vi "slider timer .vi"(6 "interval (sec)":dbl=nan, 7 "action":T1, 11 "timer ref":refnum<vi>) -> (1 "tic":bool, 2 "tic state":enum16{"knock-knock", "none"}(ring), 3 "timer out":refnum<vi>)   [LabVIEW 2015]
uses:
  countdown control.ctl
  Q - not nan -- real.vi
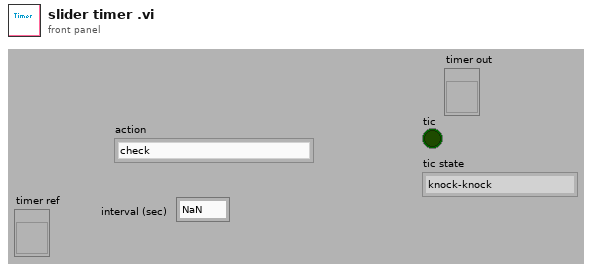
[diagram p1: front panel]
types:
  T1 = typedef "countdown control.ctl" = enum16{"check", "start", "reset cont", "stop", "reset once"}
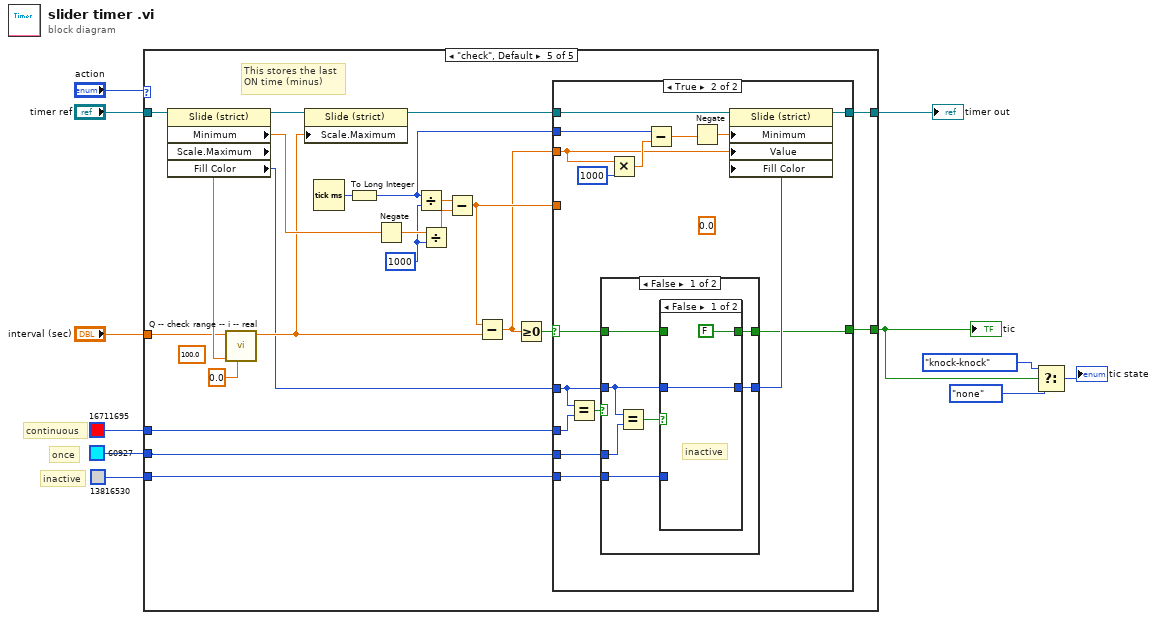
[diagram p0: block diagram]
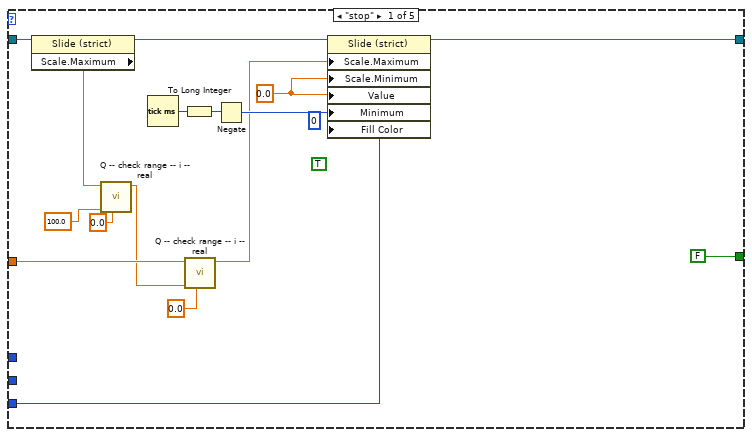
[diagram p2: hidden frame]
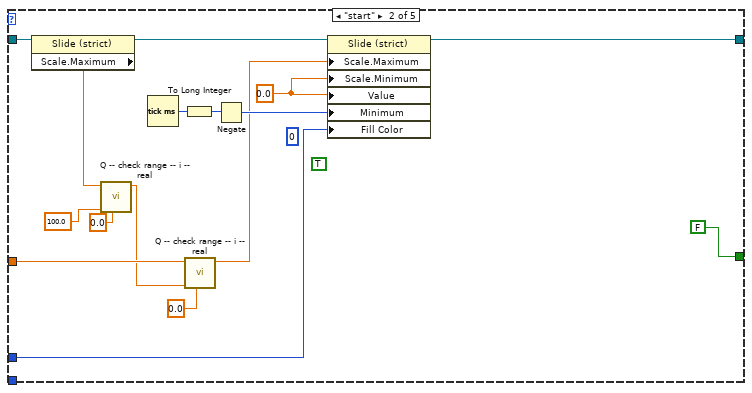
[diagram p3: hidden frame]
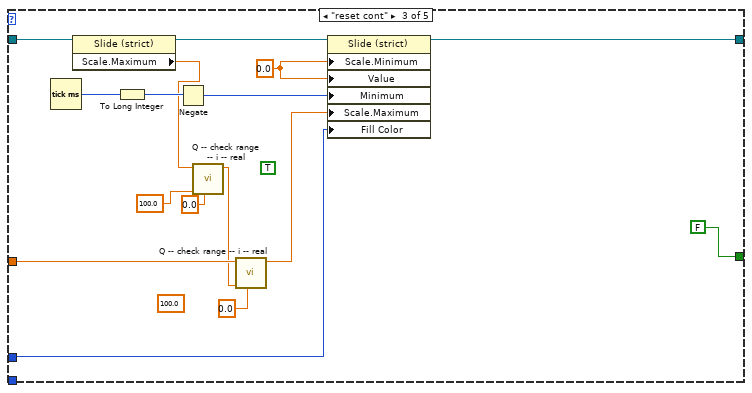
[diagram p4: hidden frame]
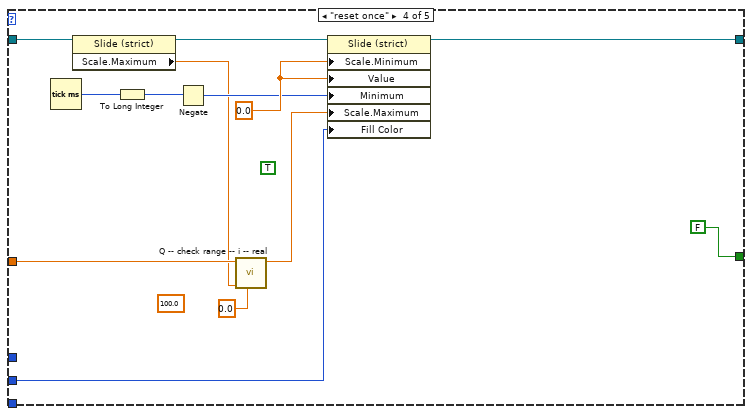
[diagram p5: hidden frame]
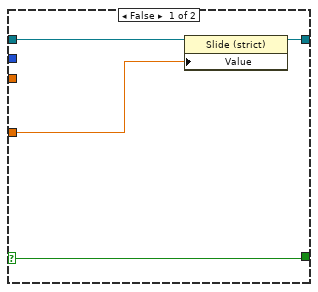
[diagram p6: hidden frame]
diagram:
  # "inactive"
  # "once"
  # "continuous"
  n1 = case shown="\"check\", Default" "action" {
    tunnel: "interval (sec)" -> [w21 w37 w50 w63 w81]
    tunnel: [FALSE FALSE FALSE FALSE w95] -> w9
    tunnel: [w25 w41 w57 w70 w91] -> w5
    tunnel: "timer ref" -> [w18 w34 w53 w66 w93]
    tunnel: u32 60927 -> [_ _ _ w60 w74]
    tunnel: u32 16711695 -> [_ w28 w48 _ w76]
    tunnel: u32 13816530 -> [w12 _ _ _ w73]
    frame "stop" {
      (unwired) u32 0 ("Fill Color")
      (unwired) TRUE
      w26 = 0.0 ("Thermometer")
      n2 = property class="Slide (strict)"(reference=w18) -> (reference out=w17:refnum<vi>, "Scale.Maximum"=w15:dbl)  [unwired: 1 in, 1 out]
      n3 = call "Q -- check range -- i -- real.vi"("lower"=0.0, "default"=100.0 ("t"), "number"=w15) -> ("number in range"=w13:dbl)  [unwired: 6 in, 2 out]
      n4 = Tick Count (ms)() -> (millisecond timer value=w23:u32)
      n5 = To Long Integer(number=w23) -> (32bit integer=w22:i32)
      n6 = call "Q -- check range -- i -- real.vi"("lower"=0.0, "default"=w13, "number"=w21) -> ("number in range"=w19:dbl)  [unwired: 6 in, 2 out]
      n7 = Negate(x=w22) -> (-x=w24:i32)
      n8 = property class="Slide (strict)"(reference=w17, "Scale.Maximum"=w19, "Scale.Minimum"=w26, "Value"=w26, "Minimum"=w24, "Fill Color"=w12) -> (reference out=w25:refnum<vi>)  [unwired: 1 in, 1 out]
    }
    frame "start" {
      (unwired) u32 0 ("Fill Color")
      (unwired) TRUE
      w42 = 0.0 ("Thermometer")
      n9 = property class="Slide (strict)"(reference=w34) -> (reference out=w33:refnum<vi>, "Scale.Maximum"=w31:dbl)  [unwired: 1 in, 1 out]
      n10 = call "Q -- check range -- i -- real.vi"("lower"=0.0, "default"=100.0 ("t"), "number"=w31) -> ("number in range"=w29:dbl)  [unwired: 6 in, 2 out]
      n11 = Tick Count (ms)() -> (millisecond timer value=w39:u32)
      n12 = To Long Integer(number=w39) -> (32bit integer=w38:i32)
      n13 = call "Q -- check range -- i -- real.vi"("lower"=0.0, "default"=w29, "number"=w37) -> ("number in range"=w35:dbl)  [unwired: 6 in, 2 out]
      n14 = Negate(x=w38) -> (-x=w40:i32)
      n15 = property class="Slide (strict)"(reference=w33, "Scale.Maximum"=w35, "Scale.Minimum"=w42, "Value"=w42, "Minimum"=w40, "Fill Color"=w28) -> (reference out=w41:refnum<vi>)  [unwired: 1 in, 1 out]
    }
    frame "reset cont" {
      (unwired) 100.0 ("t")
      (unwired) TRUE
      w58 = 0.0 ("Thermometer")
      n16 = Tick Count (ms)() -> (millisecond timer value=w55:u32)
      n17 = property class="Slide (strict)"(reference=w53) -> (reference out=w52:refnum<vi>, "Scale.Maximum"=w44:dbl)  [unwired: 1 in, 1 out]
      n18 = To Long Integer(number=w55) -> (32bit integer=w54:i32)
      n19 = Negate(x=w54) -> (-x=w56:i32)
      n20 = call "Q -- check range -- i -- real.vi"("lower"=0.0, "default"=100.0 ("t"), "number"=w44) -> ("number in range"=w45:dbl)  [unwired: 6 in, 2 out]
      n21 = call "Q -- check range -- i -- real.vi"("lower"=0.0, "default"=w45, "number"=w50) -> ("number in range"=w49:dbl)  [unwired: 6 in, 2 out]
      n22 = property class="Slide (strict)"(reference=w52, "Scale.Minimum"=w58, "Value"=w58, "Minimum"=w56, "Scale.Maximum"=w49, "Fill Color"=w48) -> (reference out=w57:refnum<vi>)  [unwired: 1 in, 1 out]
    }
    frame "reset once" {
      (unwired) 100.0 ("t")
      (unwired) TRUE
      w71 = 0.0 ("Thermometer")
      n23 = Tick Count (ms)() -> (millisecond timer value=w68:u32)
      n24 = property class="Slide (strict)"(reference=w66) -> (reference out=w65:refnum<vi>, "Scale.Maximum"=w61:dbl)  [unwired: 1 in, 1 out]
      n25 = To Long Integer(number=w68) -> (32bit integer=w67:i32)
      n26 = Negate(x=w67) -> (-x=w69:i32)
      n27 = call "Q -- check range -- i -- real.vi"("lower"=0.0, "default"=w61, "number"=w63) -> ("number in range"=w62:dbl)  [unwired: 6 in, 2 out]
      n28 = property class="Slide (strict)"(reference=w65, "Scale.Minimum"=w71, "Value"=w71, "Minimum"=w69, "Scale.Maximum"=w62, "Fill Color"=w60) -> (reference out=w70:refnum<vi>)  [unwired: 1 in, 1 out]
    }
    frame "check", Default {
      (unwired) 100.0 ("t")
      w77 = 1000
      # "This stores the last \nON time (minus)"
      n29 = property class="Slide (strict)"(reference=w93) -> (reference out=w85:refnum<vi>, "Minimum"=w87:dbl, "Scale.Maximum"=w82:dbl, "Fill Color"=w75:u32)  [unwired: 1 in, 1 out]
      n30 = call "Q -- check range -- i -- real.vi"("lower"=0.0, "default"=w82, "number"=w81) -> ("number in range"=w80:dbl)  [unwired: 6 in, 2 out]
      n31 = property class="Slide (strict)"(reference=w85, "Scale.Maximum"=w80) -> (reference out=w84:refnum<vi>)  [unwired: 1 in, 1 out]
      n32 = Tick Count (ms)() -> (millisecond timer value=w79:u32)
      n33 = To Long Integer(number=w79) -> (32bit integer=w78:i32)
      n34 = Negate(x=w87) -> (-x=w86:dbl)
      n35 = Divide(x=w78, y=w77) -> (x/y=w94:dbl)
      n36 = Divide(x=w86, y=w77) -> (x/y=w92:dbl)
      n37 = Subtract(x=w94, y=w92) -> (x-y=w90:dbl)
      n38 = Subtract(x=w90, y=w80) -> (x-y=w88:dbl)
      n39 = Greater Or Equal To 0?(x=w88) -> (x >= 0?=w89:bool)
      n40 = case shown="True" w89 {
        selector: w89 -> [w99 w102]
        tunnel: [w99 w101] -> w95
        tunnel: w90 -> [w98 _]
        tunnel: w84 -> [w96 w115]
        tunnel: w78 -> [_ w111]
        tunnel: [w97 w114] -> w91
        tunnel: w88 -> [_ w108]
        tunnel: w75 -> [_ w105]
        tunnel: w76 -> [_ w107]
        tunnel: w74 -> [_ w103]
        tunnel: w73 -> [_ w100]
        frame False {
          n41 = property class="Slide (strict)"(reference=w96, "Value"=w98) -> (reference out=w97:refnum<vi>)  [unwired: 1 in, 1 out]
        }
        frame True {
          (unwired) 0.0 ("Value")
          n42 = Equal?(x=w105, y=w107) -> (x = y?=w106:bool)
          n43 = case shown="False" w106 {
            tunnel: [w118 w128] -> w104
            tunnel: w105 -> [w116 w128]
            tunnel: w103 -> [w122 _]
            tunnel: w102 -> [w120 w127]
            tunnel: [w119 w127] -> w101
            tunnel: w100 -> [w117 _]
            frame False {
              n44 = Equal?(x=w116, y=w122) -> (x = y?=w121:bool)
              n45 = case shown="False" w121 {
                tunnel: [FALSE w126] -> w119
                tunnel: w120 -> [_ w126]
                tunnel: [w123 w125] -> w118
                tunnel: w117 -> [_ w125]
                tunnel: w116 -> [w123 _]
                frame False {
                  # "inactive"
                }
                frame True {
                  # "once"
                }
              }
            }
            frame True {
              # "continuous"
            }
          }
          n46 = Multiply(x=w108, y=1000) -> (x*y=w112:dbl)
          n47 = Subtract(x=w111, y=w112) -> (x-y=w109:dbl)
          n48 = Negate(x=w109) -> (-x=w110:dbl)
          n49 = property class="Slide (strict)"(reference=w115, "Minimum"=w110, "Value"=w108, "Fill Color"=w104) -> (reference out=w114:refnum<vi>)  [unwired: 1 in, 1 out]
        }
      }
    }
  }
  "tic" <- w9
  "timer out" <- w5
  n50 = Select(t=enum16{"knock-knock", "none"}."knock-knock" ("state"), s=w9, f=enum16{"knock-knock", "none"}."none" ("state")) -> (s? t:f=→"tic state":enum16{"knock-knock", "none"})
